vi "splash_screen_launcher_v1.0.vi"(8 "error in (no error)":errorcluster, 9 "transparency_rate(ms)":i32=25, 10 "close_delay(sec)":dbl=5.0, 11 "message in":string="Loading DAQ resources...") -> (0 "error out":errorcluster)   [LabVIEW 2025]
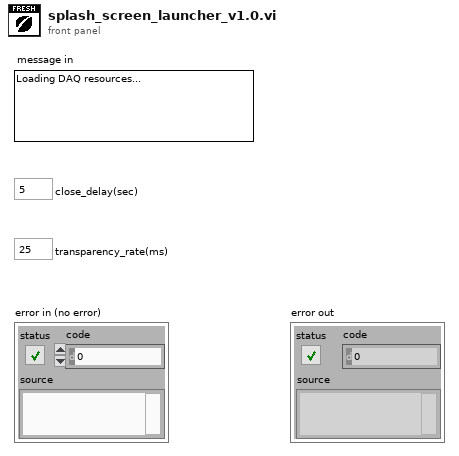
[diagram p1: front panel]
types:
  T1 = enum32{"Invalid", "Standard", "Closed", "Hidden", "Minimized", "Maximized"}
  T2 = enum32{"Bad", "Idle", "Run top level", "Running"}
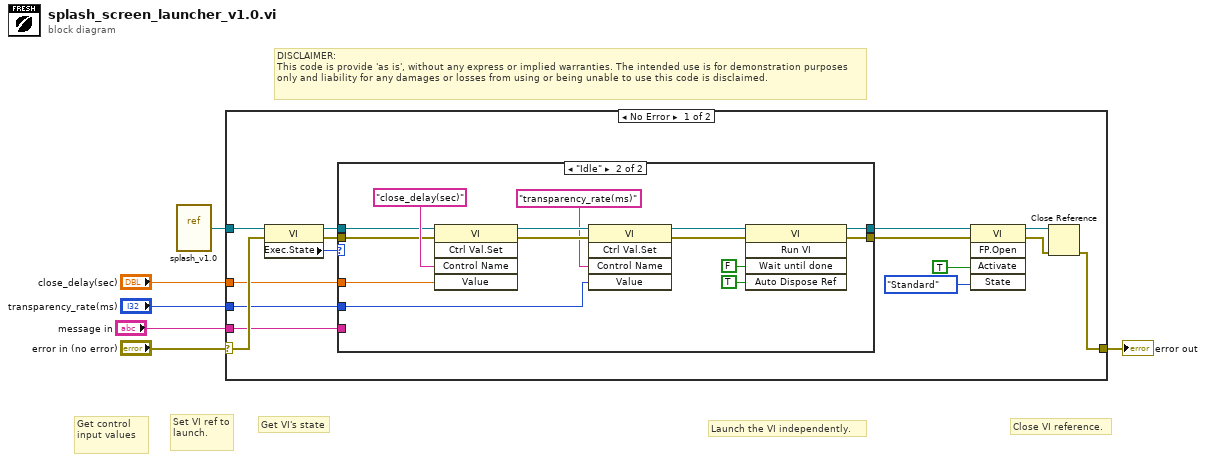
[diagram p0: block diagram]
diagram:
  # "Close VI reference."
  # "Launch the VI independently."
  # "Get VI's state"
  # "Set VI ref to launch."
  # "Get control input values"
  # "DISCLAIMER:\nThis code is provide 'as is', without any express or implied warranties. The intended use is for demonstration purposes only and liability for any damages or losses from using or being unable to use this code is disclaimed."
  n1 = vi-ref "splash_v1.0.vi"() -> (w6:refnum<vi>)
  n2 = case shown="No Error" "error in (no error)" {
    selector: "error in (no error)" -> [w17 w38]
    tunnel: w6 -> [w16 _]
    tunnel: [w18 w38] -> w4
    tunnel: "close_delay(sec)" -> [w15 _]
    tunnel: "transparency_rate(ms)" -> [w14 _]
    tunnel: "message in" -> [w13 _]
    frame No Error {
      n3 = property class="VI"(reference=w16, error in=w17) -> (reference out=w20:refnum<vi>, error out=w19:errorcluster, "Exec.State"=w21:T2)
      n4 = case shown="\"Idle\"" w21 {
        tunnel: w20 -> [w22 w28]
        tunnel: w19 -> [w23 w27]
        tunnel: [w22 w35] -> w10
        tunnel: [w23 w34] -> w9
        tunnel: w15 -> [_ w25]
        tunnel: w14 -> [_ w24]
        tunnel: w13 -> [_ _]
        frame Default {
        }
        frame "Idle" {
          n5 = invoke class="VI" method="Ctrl Val.Set"(reference=w28, error in=w27, "Control Name"="close_delay(sec)", "Value"=w25) -> (reference out=w32:refnum<vi>, error out=w33:errorcluster)  [unwired: 1 in, 3 out]
          n6 = invoke class="VI" method="Ctrl Val.Set"(reference=w32, error in=w33, "Control Name"="transparency_rate(ms)", "Value"=w24) -> (reference out=w29:refnum<vi>, error out=w26:errorcluster)  [unwired: 1 in, 3 out]
          n7 = invoke class="VI" method="Run VI"(reference=w29, error in=w26, "Wait until done"=FALSE ("Wait Until Done"), "Auto Dispose Ref"=TRUE ("Auto Dispose Reference")) -> (reference out=w35:refnum<vi>, error out=w34:errorcluster)  [unwired: 1 in, 3 out]
        }
      }
      n8 = invoke class="VI" method="FP.Open"(reference=w10, error in=w9, "Activate"=TRUE ("Activate?"), "State"=T1."Standard") -> (reference out=w7:refnum<vi>, error out=w8:errorcluster)  [unwired: 1 in, 3 out]
      n9 = Close Reference(reference=w7, error in (no error)=w8) -> (error out=w18:errorcluster)
    }
    frame Error {
    }
  }
  "error out" <- w4
